vi "Main.vi"(11 "Module Admin":refnum<class "Delacor_lib_QMH_Module Admin.lvclass">) -> ()   [LabVIEW 2020, in "Acquisition.lvlib"]
doc: "This template is based off of the Queued Message Handler design pattern and the Queued Message Handler project template that ships with LabVIEW.\n\nThe main difference is that the queue is private to this module and communication between modules is performed via Broadcast and Request events.\n\nRequest events are wrapped in public API methods and are handled in the Event Handling Loop (EHL) of this VI. Any module can register for Broadcast events sent by this module. The EHL generates messages based on user interface actions.\n\nThe Message Handling Loop (MHL) processes messages generated by the EHL, or by other messages. The messages are string values, so new messages can be added easily to the Message Cases case structure in the MHL. Each message cluster can also provide an optional value for Message Data, which is a variant that can be converted to whatever message-specific data is required.\n_____\nBased on Delacor QMH Project Template 6.0.0.89."
uses:
  Acquisition.lvlib
  <vilib>/Delacor/Delacor QMH/Libraries/Module Admin_class/Delacor_lib_QMH_Module Admin.lvclass
  Module Data--cluster.ctl
  DigitalConfig--cluster.ctl
  AnalogConfig--cluster.ctl
  Stop Argument--cluster.ctl
  <vilib>/Delacor/Delacor QMH/Libraries/Message Queue_class/Delacor_lib_QMH_Message Queue.lvclass/Delacor_lib_QMH_Message Queue.ctl
  <vilib>/Delacor/Delacor QMH/Libraries/Module Admin_class/Delacor_lib_QMH_Module Admin.lvclass/Delacor_lib_QMH_Module Admin.ctl
  Start Acquistion Argument--cluster.ctl
  Set Secuence Argument--cluster.ctl
  <vilib>/Utility/miscctls.llb/LVPointTypeDef.ctl
  <vilib>/DAQmx/read.llb/DAQmx Read (Digital 1D U8 NChan 1Samp).vi
  <vilib>/DAQmx/read.llb/DAQmx Read (Digital 1D Bool NChan 1Samp 1Line).vi
  <vilib>/DAQmx/read.llb/DAQmx Read (Analog 1D Wfm NChan NSamp).vi
  <vilib>/Delacor/Delacor QMH/Libraries/Message Queue_class/Delacor_lib_QMH_Enqueue Message (Single).vi
  <vilib>/Delacor/Delacor QMH/Libraries/Module Admin_class/Delacor_lib_QMH_Get External Launch.vi
  <vilib>/DAQmx/miscellaneous.llb/DAQmx Fill In Error Info.vi
  <vilib>/Utility/error.llb/Error Cluster From Error Code.vi
  <vilib>/ErrorRing/Error Ring.xnode
  <vilib>/Delacor/Delacor QMH/Libraries/Message Queue_class/Delacor_lib_QMH_Message Queue.lvclass
panel:
  out "element":string
  out "error out":errorcluster
  out "Status":string
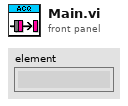
[diagram p1: front panel]
types:
  T1 = typedef "Acquisition.lvlib/Request Events--cluster.ctl" = cluster{"Stop Module":refnum<user-event>, "Show Panel":refnum<user-event>, "Hide Panel":refnum<user-event>, "Get Module Execution Status":refnum<user-event>, "Show Diagram":refnum<user-event>, "Start Acquistion":refnum<user-event>, "WakeUp Digital HL":refnum<user-event>, "WakeUp Analog HL":refnum<user-event>, "Put Analog HL to Sleep":refnum<user-event>, "Put Digital HL to Sleep":refnum<user-event>, "Set Secuence":refnum<user-event>}
  T2 = typedef "Acquisition.lvlib/Module Data--cluster.ctl" = cluster{"Status":string, "DigitalConfig":T3, "AnalogConfig":T4, "ID Max":i32, "Secuence":string[][]}
  T3 = typedef "DigitalConfig--cluster.ctl" = cluster{"Ports/Pins":enum16{"PORTS", "PINS"}, "AcqTime":dbl, "AcqFrecuency":dbl, "Port Digitales":tag[], "Pins":tag[]}
  T4 = typedef "AnalogConfig--cluster.ctl" = cluster{"AcqTime":dbl, "FSamples":dbl, "NSamples":dbl, "Channels":tag[]}
  T5 = enum32{"invalid lock state", "Not Locked", "Locked (No Password)", "Password-protected"}
  T6 = typedef "Acquisition.lvlib/Stop Argument--cluster.ctl" = cluster{"Origin":string, "Exit via Stop Module Req?":bool, "Wait for Module to stop?":bool}
  T7 = typedef "Acquisition.lvlib/Start Acquistion Argument--cluster.ctl" = cluster{"Boolean":bool}
  T8 = typedef "Acquisition.lvlib/Set Secuence Argument--cluster.ctl" = cluster{"ID Max":i32, "Secuence":string[][]}
  T9 = typedef "LVPointTypeDef.ctl" = cluster{"Horizontal":i16, "Vertical":i16}
  T10 = enum32{"Invalid", "Standard", "Closed", "Hidden", "Minimized", "Maximized"}
  T11 = typedef "AcqType--enum.ctl" = enum16{"Digital", "Analog"}
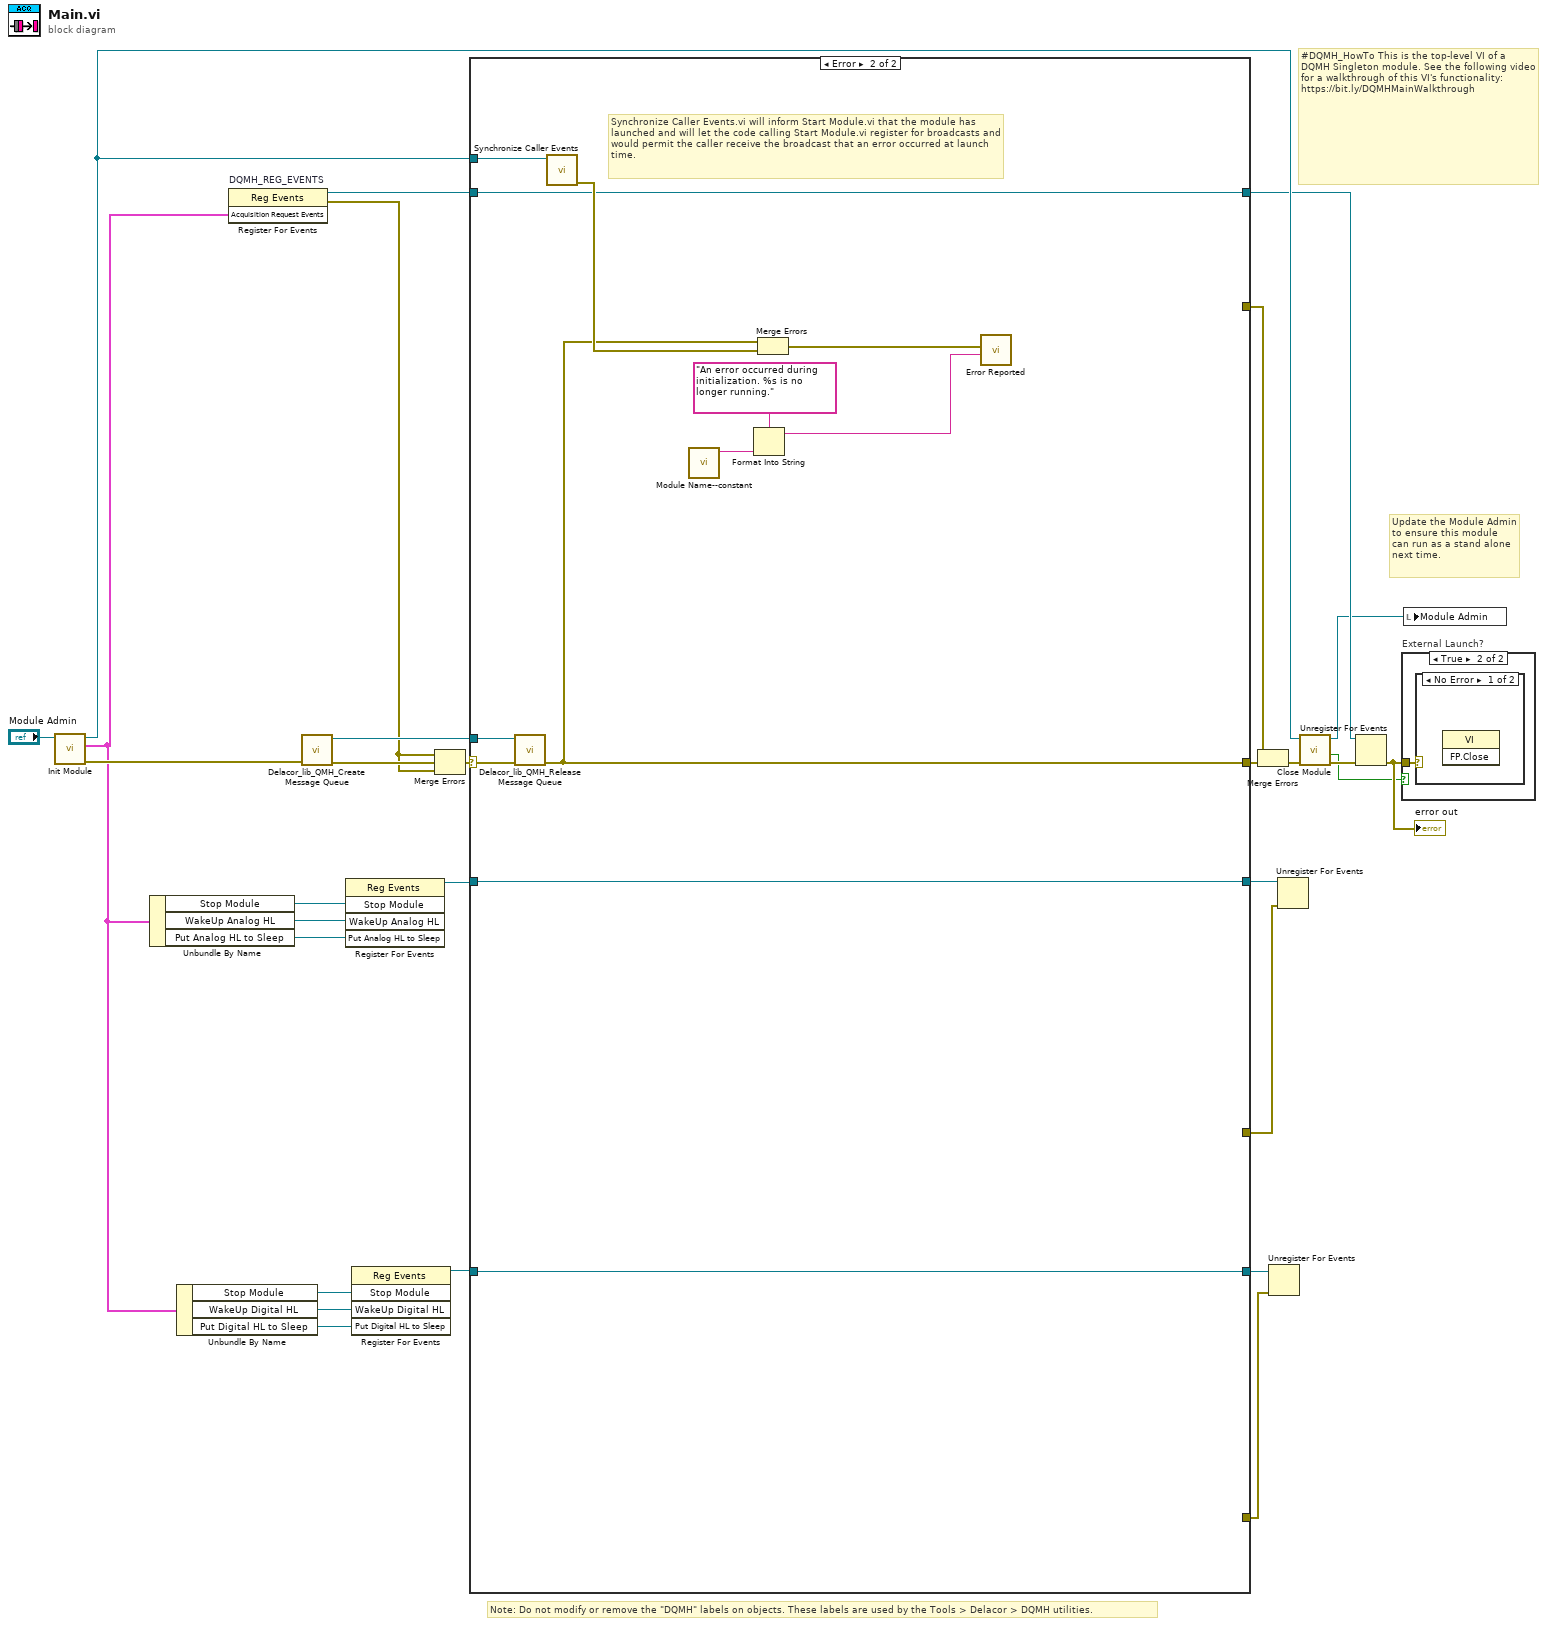
[diagram p0: block diagram]
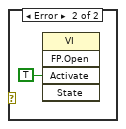
[diagram p3: hidden frame]
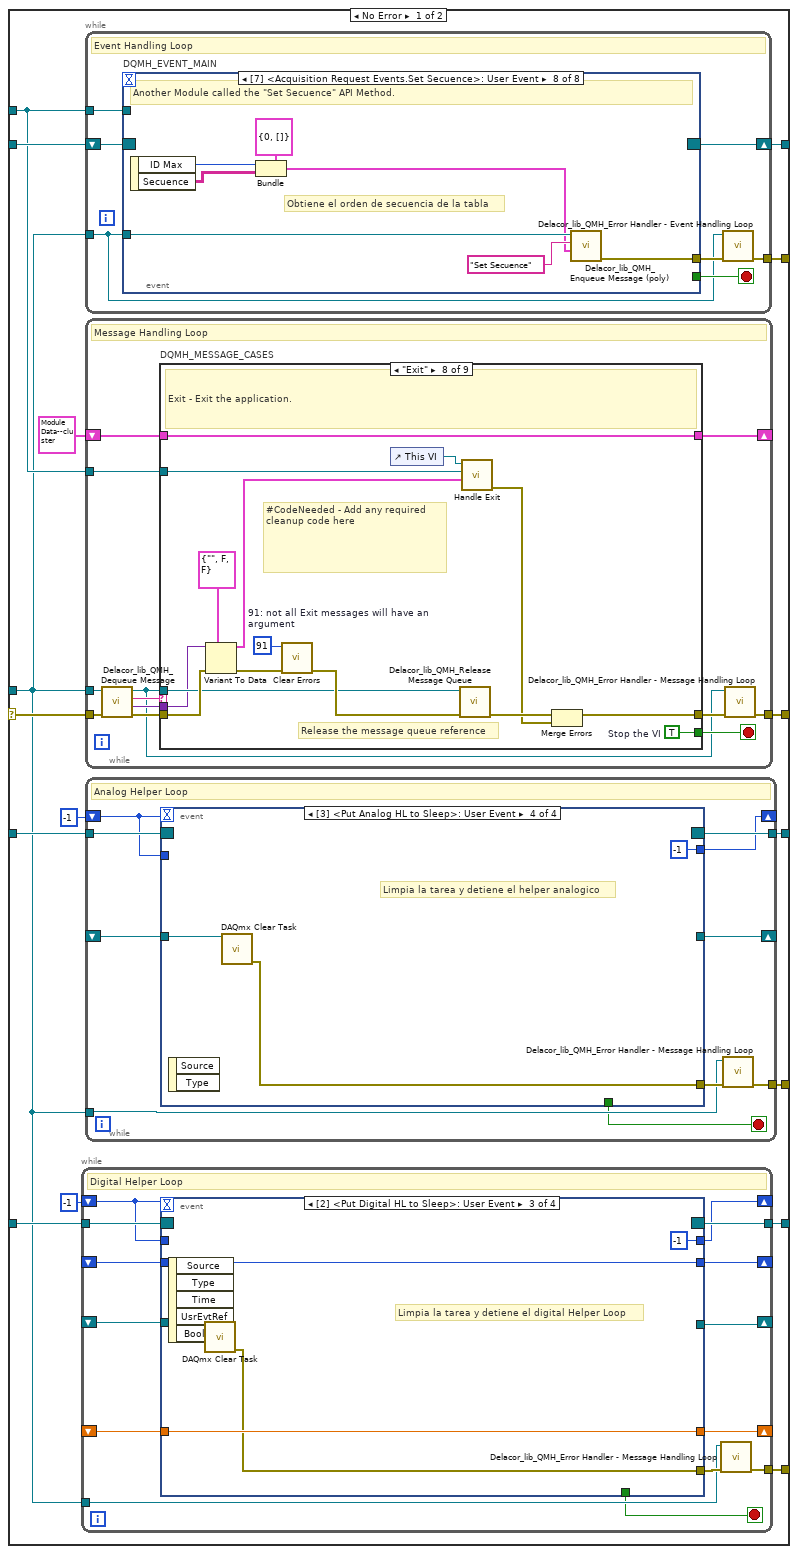
[diagram p4: hidden frame]
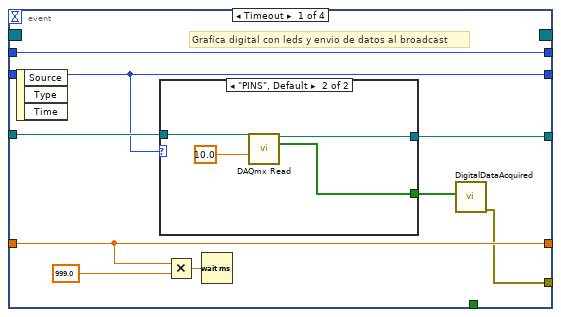
[diagram p5: hidden frame]
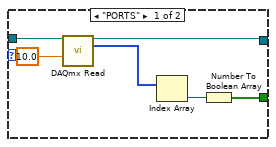
[diagram p6: hidden frame]
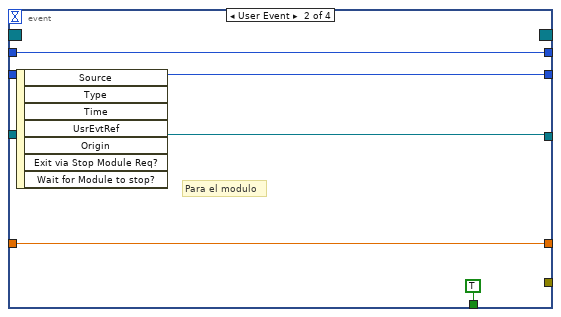
[diagram p7: hidden frame]
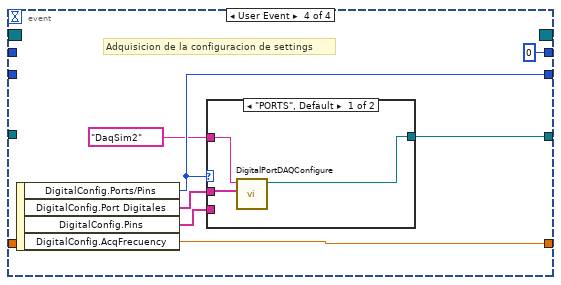
[diagram p8: hidden frame]
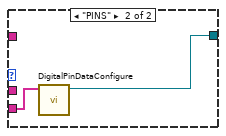
[diagram p9: hidden frame]
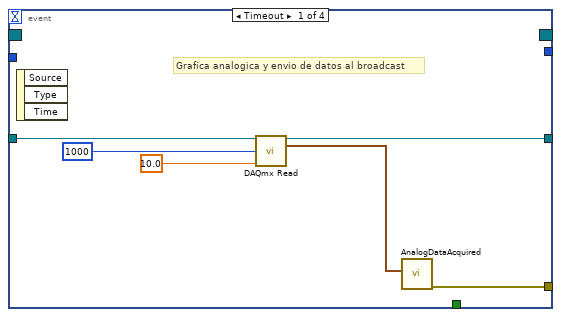
[diagram p10: hidden frame]
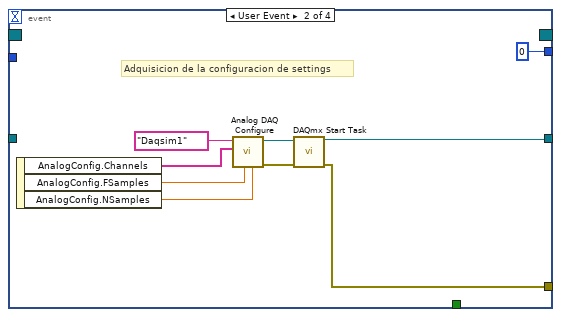
[diagram p11: hidden frame]
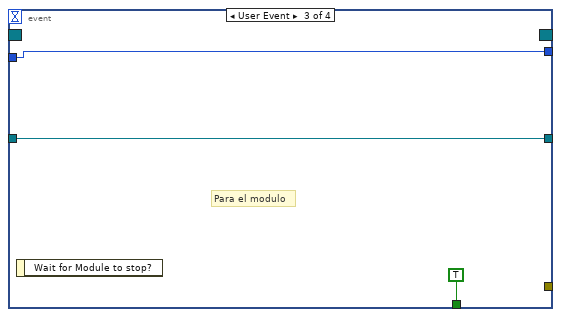
[diagram p12: hidden frame]
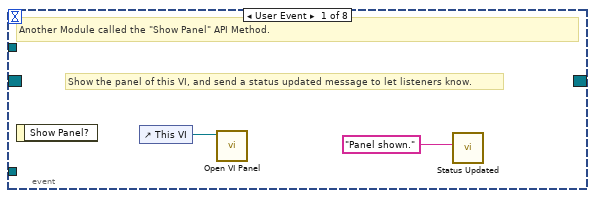
[diagram p13: hidden frame]
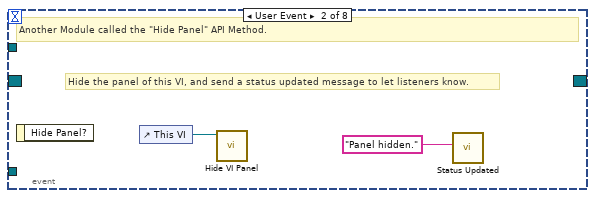
[diagram p14: hidden frame]
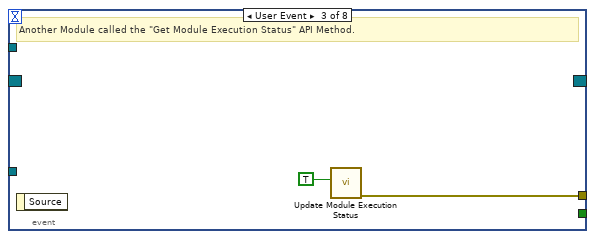
[diagram p15: hidden frame]
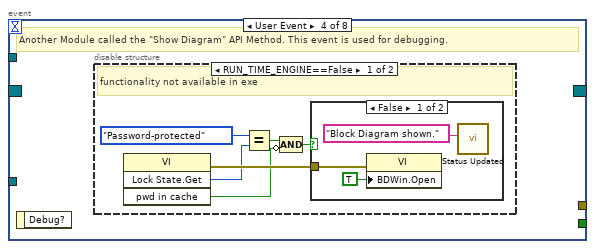
[diagram p16: hidden frame]
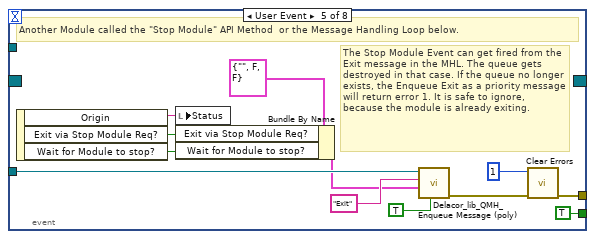
[diagram p19: hidden frame]
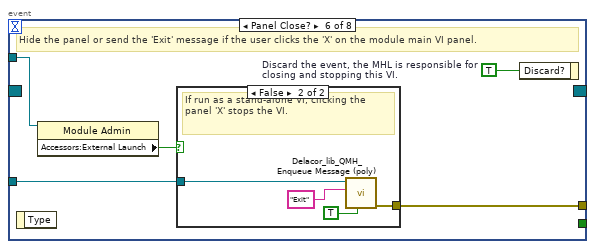
[diagram p20: hidden frame]
diagram:
  # "#DQMH_HowTo This is the top-level VI of a DQMH Singleton module. See the following video for a walkthrough of this VI's functionality: https://bit.ly/DQMHMainWalkthrough"
  # "Note: Do not modify or remove the \"DQMH\" labels on objects. These labels are used by the Tools > Delacor > DQMH utilities."
  # "Update the Module Admin to ensure this module can run as a stand alone next time."
  n1 = call "Init Module.vi"("Singleton Module Admin in"="Module Admin") -> ("error out"=w28:errorcluster, "Acquisition Request Events"=w7:T1, "Singleton Module Admin out"=w21:refnum<class "Delacor_lib_QMH_Module Admin.lvclass">)  [unwired: 8 in]
  n2 = Unbundle By Name(w7) -> ("Stop Module"=w10:refnum<user-event>, "WakeUp Analog HL"=w8:refnum<user-event>, "Put Analog HL to Sleep"=w9:refnum<user-event>)
  n3 = Unbundle By Name(w7) -> ("Stop Module"=w6:refnum<user-event>, "WakeUp Digital HL"=w5:refnum<user-event>, "Put Digital HL to Sleep"=w4:refnum<user-event>)
  n4 = register-events "DQMH_REG_EVENTS"(w7) -> (reference out=w19:refnum<event-registration>, error out=w1:errorcluster)  [unwired: 2 in]
  n5 = call <vilib>:"Delacor_lib_QMH_Create Message Queue.vi"("error in"=w28) -> ("error out"=w23:errorcluster, "Message Queue"=w18:refnum<class "Delacor_lib_QMH_Message Queue.lvclass">)  [unwired: 9 in]
  n6 = register-events(w10, w8, w9) -> (reference out=w12:refnum<event-registration>)  [unwired: 2 in, 1 out]
  n7 = register-events(w6, w5, w4) -> (reference out=w11:refnum<event-registration>)  [unwired: 2 in, 1 out]
  n8 = Merge Errors(w1, w23, w1) -> (w22:errorcluster)
  n9 = case shown="Error" w22 {
    selector: w22 -> [w43 w319]
    tunnel: [w45 w318] -> w29
    tunnel: [w42 w324] -> w20
    tunnel: w19 -> [w40 w324]
    tunnel: w18 -> [w30 w317]
    tunnel: [w44 _] -> w26
    tunnel: w21 -> [w39 w320]
    tunnel: [w38 w316] -> w14
    tunnel: [w37 w315] -> w13
    tunnel: w12 -> [w36 w316]
    tunnel: w11 -> [w35 w315]
    tunnel: [w32 _] -> w3
    tunnel: [w31 _] -> w2
    frame No Error {
      n10 = while {
        tunnel: [w59] -> w37
        tunnel: w35 -> [w58]
        shift-right: [w49] -> _
        shift-left: -1 -> [w57]
        tunnel: [w56] -> w31
        tunnel: w30 -> [w54]
        shift-right: [w52] -> _
        shift-left: _ -> [w53]
        shift-right: [w50] -> _
        shift-left: _ -> [w51]
        shift-right: [w48] -> _
        shift-left: _ -> [w47]
        stop <- w46 stop-if-true
        # "Digital Helper Loop"
        n11 = event shown="[2] <Put Digital HL to Sleep>: User Event" {
          selector: w58 -> [_ _ _ _]
          dyn-events: [_ _ _ _] -> w59
          timeout: w57 -> [_ _ _ _]
          tunnel: w57 -> [w65 w82 _ _]
          tunnel: [w61 _ w84 _] -> w55
          tunnel: w53 -> [w68 w81 w85 _]
          tunnel: [w67 w81 _ w90] -> w52
          tunnel: w51 -> [w63 w80 w86 _]
          tunnel: [w63 w80 w86 w95] -> w50
          tunnel: [w65 w82 -1 0] -> w49
          tunnel: [w60 w83 w88 w93] -> w48
          tunnel: w47 -> [w60 w83 w88 _]
          tunnel: [_ TRUE _ _] -> w46
          event Timeout {
            # "Grafica digital con leds y envio de datos al broadcast"
            n12 = event-data() -> ()  [unwired: 1 in, 3 out]
            n13 = case shown="\"PINS\", Default" w60 {
              tunnel: w68 -> [w74 w78]
              tunnel: [w73 w77] -> w67
              tunnel: [w70 w76] -> w66
              frame "PORTS" {
                n14 = call-poly <vilib>:"DAQmx Read.vi"("task/channels in"=w74, "timeout"=10.0) -> ("task out"=w73:refnum<k21>, "data"=w72:u8[])  [unwired: 11 in, 1 out]
                n15 = Index Array(array=w72) -> (element=w71:u8)  [unwired: 1 in]
                n16 = Number To Boolean Array(number=w71) -> (Boolean array=w70:bool[])
              }
              frame "PINS", Default {
                n17 = call-poly <vilib>:"DAQmx Read.vi"("task/channels in"=w78, "timeout"=10.0) -> ("task out"=w77:refnum<k21>, "data"=w76:bool[])  [unwired: 11 in, 1 out]
              }
            }
            n18 = Multiply(x=w63, y=999.0) -> (x*y=w64:dbl)
            n19 = Wait (ms)(milliseconds to wait=w64) -> ()  [unwired: 1 out]
            n20 = call "DigitalDataAcquired.vi"("DigitalData"=w66) -> ("error out"=w61:errorcluster)  [unwired: 10 in]
          }
          event User Event {
            # "Para el modulo"
            n21 = event-data() -> ()  [unwired: 1 in, 7 out]
          }
          event User Event {
            # "Limpia la tarea y detiene el digital Helper Loop"
            n22 = event-data() -> ()  [unwired: 1 in, 5 out]
            n23 = call <vilib>:"DAQmx Clear Task.vi"("task in"=w85) -> ("error out"=w84:errorcluster)  [unwired: 14 in]
          }
          event User Event {
            # "Adquisicion de la configuracion de settings"
            n24 = event-data() -> ("DigitalConfig.Ports/Pins"=w93:enum16{"PORTS", "PINS"}, "DigitalConfig.Port Digitales"=w92:tag[], "DigitalConfig.Pins"=w89:tag[], "DigitalConfig.AcqFrecuency"=w95:dbl)  [unwired: 1 in]
            n25 = case shown="\"PORTS\", Default" w93 {
              tunnel: w92 -> [w98 _]
              tunnel: tag "DaqSim2" ("DAQmx Device Digital") -> [w97 _]
              tunnel: [w96 w100] -> w90
              tunnel: w89 -> [_ w99]
              frame "PORTS", Default {
                n26 = call "DigitalPortDAQConfigure.vi"("Port Digitales"=w98, "DAQmx Device Digital"=w97) -> ("task out"=w96:refnum<k21>)  [unwired: 8 in, 1 out]
              }
              frame "PINS" {
                n27 = call "DigitalPinDataConfigure.vi"("Pins"=w99) -> ("task out"=w100:refnum<k21>)  [unwired: 9 in, 1 out]
              }
            }
          }
        }
        n28 = call-dynamic "Delacor_lib_QMH_Error Handler - Message Handling Loop.vi"("error in"=w55, "Message Queue in"=w54) -> ("dup error in"=w56:errorcluster)  [unwired: 8 in, 1 out]
      }
      n29 = while {
        tunnel: w30 -> [w132]
        shift-right: [w135] -> w42
        shift-left: w40 -> [w136]
        tunnel: [w137] -> w44
        tunnel: w39 -> [w133]
        stop <- w134 stop-if-true
        # "Event Handling Loop"
        n30 = event "DQMH_EVENT_MAIN" shown="[7] <Acquisition Request Events.Set Secuence>: User Event" {
          selector: w136 -> [_ _ _ _ _ _ _ _]
          dyn-events: [_ _ _ _ _ _ _ _] -> w135
          timeout: _ -> [_ _ _ _ _ _ _ _]
          tunnel: [_ _ _ _ TRUE ("Discard?") _ _ _] -> w134
          tunnel: w132 -> [_ _ _ _ w161 w168 w181 w188]
          tunnel: [_ _ w144 _ w164 w170 w176 w182] -> w138
          tunnel: w133 -> [_ _ _ _ _ w167 _ _]
          event User Event {
            # "Show the panel of this VI, and send a status updated message to let listeners know."
            # "Another Module called the \"Show Panel\" API Method."
            n31 = event-data() -> ()  [unwired: 1 in, 1 out]
            n32 = control-ref of="This VI"() -> (w140:refnum<vi>)
            n33 = call "Open VI Panel.vi"("VI"=w140) -> ()  [unwired: 10 in, 1 out]
            n34 = call "Status Updated.vi"("Status"="Panel shown." ("format string")) -> ()  [unwired: 10 in, 1 out]
          }
          event User Event {
            # "Hide the panel of this VI, and send a status updated message to let listeners know."
            # "Another Module called the \"Hide Panel\" API Method."
            n35 = event-data() -> ()  [unwired: 1 in, 1 out]
            n36 = control-ref of="This VI"() -> (w142:refnum<vi>)
            n37 = call "Hide VI Panel.vi"("VI"=w142) -> ()  [unwired: 10 in, 1 out]
            n38 = call "Status Updated.vi"("Status"="Panel hidden." ("format string")) -> ()  [unwired: 10 in, 1 out]
          }
          event User Event {
            # "Another Module called the \"Get Module Execution Status\" API Method."
            n39 = event-data() -> ()  [unwired: 1 in, 1 out]
            n40 = call "Update Module Execution Status.vi"("Running?"=TRUE) -> ("error out"=w144:errorcluster)  [unwired: 10 in]
          }
          event User Event {
            # "Another Module called the \"Show Diagram\" API Method. This event is used for debugging."
            n41 = event-data() -> ()  [unwired: 1 in, 1 out]
            n42 = disable-structure shown="RUN_TIME_ENGINE==False" {
              frame condition #0 (active) {
                # "functionality not available in exe"
                n43 = invoke class="VI" method="Lock State.Get"() -> (error out=w150:errorcluster, "Get Lock State"=w149:T5, "pwd in cache"=w146:bool)  [unwired: 4 in, 1 out]
                n44 = Equal?(x=T5."Password-protected", y=w149) -> (x = y?=w147:bool)
                n45 = Compound Arithmetic op=AND(w147, invert w146) -> (w145:bool)
                n46 = case shown="False" w145 {
                  tunnel: w150 -> [w153 _]
                  frame False {
                    n47 = property class="VI"(error in=w153, "BDWin.Open"=TRUE ("Block Diagram Window:Open")) -> ()  [unwired: 1 in, 2 out]
                    n48 = call "Status Updated.vi"("Status"="Block Diagram shown." ("format string")) -> ()  [unwired: 10 in, 1 out]
                  }
                  frame True {
                    # "Password-protected VI, and the password is not in the cache. Do not show the diagram."
                  }
                }
              }
              frame condition #1 {
              }
            }
          }
          event User Event {
            # "The Stop Module Event can get fired from the Exit message in the MHL. The queue gets destroyed in that case. If the queue no longer exists, the Enqueue Exit as a priority message will return error 1. It is safe to ignore, because the module is already exiting."
            # "Another Module called the \"Stop Module\" API Method  or the Message Handling Loop below."
            n49 = event-data() -> ("Origin"=w160:string, "Exit via Stop Module Req?"=w156:bool, "Wait for Module to stop?"=w155:bool)  [unwired: 1 in]
            n50 = local write "Status"(w160) -> ()
            n51 = Bundle By Name(cluster=T6 {"Origin"="", "Exit via Stop Module Req?"=FALSE, "Wait for Module to stop?"=FALSE} ("Stop Argument"), "Exit via Stop Module Req?"=w156, "Wait for Module to stop?"=w155) -> (w154:T6)
            n52 = call-poly <vilib>:"Delacor_lib_QMH_Enqueue Message (poly).vi"("Priority Message? (F)"=TRUE, "Message Data"=w154, "Message"="Exit", "Message Queue in"=w161) -> ("error out"=w165:errorcluster)  [unwired: 6 in, 1 out]
            n53 = call <vilib>:"Clear Errors.vi"("error in (no error)"=w165, "specific error code to clear (0: all)"=1) -> ("error out"=w164:errorcluster)  [unwired: 4 in, 1 out]
          }
          event Panel Close? {
            w169 = TRUE  # Discard the event, the MHL is responsible for closing and stopping this VI.
            # "Hide the panel or send the 'Exit' message if the user clicks the 'X' on the module main VI panel."
            n54 = event-data() -> ()  [unwired: 1 in, 1 out]
            n55 = property class="Module Admin"(reference=w167) -> ("Accessors:External Launch"=w166:bool)  [unwired: 1 in, 2 out]
            n56 = case shown="False" w166 {
              tunnel: w168 -> [_ w174]
              tunnel: [_ w175] -> w170
              frame True {
                # "If externally launched, clicking the 'X' hides the panel, but doesn't close it."
                n57 = control-ref of="This VI"() -> (w171:refnum<vi>)
                n58 = call "Hide VI Panel.vi"("VI"=w171) -> ()  [unwired: 10 in, 1 out]
              }
              frame False {
                # "If run as a stand-alone VI, clicking the panel 'X' stops the VI."
                n59 = call-poly <vilib>:"Delacor_lib_QMH_Enqueue Message (poly).vi"("Priority Message? (F)"=TRUE, "Message"="Exit", "Message Queue in"=w174) -> ("error out"=w175:errorcluster)  [unwired: 7 in, 1 out]
              }
            }
            n60 = event-data("Discard?"=w169) -> ()  [unwired: 1 in, 1 out]
          }
          event User Event {
            # "Another Module called the \"Start Acquistion\" API Method."
            n61 = event-data() -> ("Boolean"=w177:bool)  [unwired: 1 in]
            n62 = Bundle(cluster=T7 {"Boolean"=FALSE} ("Start Acquistion Argument"), "Boolean"=w177) -> (w178:T7)
            n63 = call-poly <vilib>:"Delacor_lib_QMH_Enqueue Message (poly).vi"("Message Data"=w178, "Message"="Start Acquistion", "Message Queue in"=w181) -> ("error out"=w176:errorcluster)  [unwired: 7 in, 1 out]
          }
          event User Event {
            # "Obtiene el orden de secuencia de la tabla"
            # "Another Module called the \"Set Secuence\" API Method."
            n64 = event-data() -> ("ID Max"=w184:i32, "Secuence"=w183:string[][])  [unwired: 1 in]
            n65 = Bundle(cluster=T8 {"ID Max"=0, "Secuence"=[]} ("Set Secuence Argument"), "ID Max"=w184, "Secuence"=w183) -> (w185:T8)
            n66 = call-poly <vilib>:"Delacor_lib_QMH_Enqueue Message (poly).vi"("Message Data"=w185, "Message"="Set Secuence", "Message Queue in"=w188) -> ("error out"=w182:errorcluster)  [unwired: 7 in, 1 out]
          }
        }
        n67 = call-dynamic "Delacor_lib_QMH_Error Handler - Event Handling Loop.vi"("error in"=w138, "Message Queue in"=w132) -> ("dup error in"=w137:errorcluster)  [unwired: 8 in, 1 out]
      }
      n68 = while {
        tunnel: w30 -> [w191]
        shift-right: [w195] -> _
        shift-left: T2 {"Status"="", "DigitalConfig"={"Ports/Pins"=enum."PORTS", "AcqTime"=0.0, "AcqFrecuency"=0.0, "Port Digitales"=[], "Pins"=[]}, "AnalogConfig"={"AcqTime"=0.0, "FSamples"=0.0, "NSamples"=0.0, "Channels"=[]}, "ID Max"=0, "Secuence"=[]} ("Data Cluster") -> [w196]
        tunnel: w43 -> [w199]
        tunnel: [w197] -> w45
        tunnel: w39 -> [w189]
        stop <- w194 stop-if-true
        # "Message Handling Loop"
        n69 = call-dynamic "Delacor_lib_QMH_Dequeue Message.vi"("error in"=w199, "Message Queue in"=w191) -> ("error out"=w198:errorcluster, "Message Data"=w192:variant, "Message"=w193:string, "Message Queue out"=w190:refnum<class "Delacor_lib_QMH_Message Queue.lvclass">)  [unwired: 6 in]
        n70 = case "DQMH_MESSAGE_CASES" shown="\"Exit\"" w193 {
          selector: w193 -> [_ _ _ _ _ _ _ _ w302]
          tunnel: w190 -> [_ _ _ _ _ _ w272 w294 _]
          tunnel: w198 -> [w218 w222 w228 w264 w267 w269 w279 w300 w304]
          tunnel: [w216 w222 w228 w263 w266 w269 w275 w297 w305] -> w200
          tunnel: w196 -> [w207 w221 w227 w259 w265 w268 w274 w293 w303]
          tunnel: [w206 w221 w227 w256 w265 w268 w274 w293 w303] -> w195
          tunnel: [_ _ _ _ _ _ _ w292 _] -> w194
          tunnel: w192 -> [_ _ _ w262 _ _ w273 w291 _]
          tunnel: w189 -> [w208 _ _ _ _ _ w271 w286 _]
          frame "Initialize" {
            w202 = "Initial Message" ("Initial Message")
            # "#CodeNeeded - Initialize the appearance of the front panel."
            # "#CodeNeeded - Initialize your state data here."
            # "Initialize - Any operation that needs to be done before the module can receive messages. Synchronize Caller Events.vi will inform Start Module.vi that the module has launched and is ready to receive messages. Module Did Init.vi will broadcast that the module initialized."
            n71 = call "Synchronize Caller Events.vi"("error in (no error)"=w218, "Singleton Module Admin in"=w208) -> ("error out"=w217:errorcluster, "Singleton Module Admin out"=w203:refnum<class "Delacor_lib_QMH_Module Admin.lvclass">)  [unwired: 8 in]
            n72 = property class="Module Admin"(reference=w203) -> ("Accessors:External Launch"=w212:bool)  [unwired: 1 in, 2 out]
            n73 = Select(t=T10."Hidden" ("State"), s=w212, f=T10."Standard" ("State")) -> (s? t:f=w209:T10)
            n74 = call "Module Name--constant.vi"() -> ("Module Name"=w215:string)  [unwired: 11 in]
            n75 = property class="VI"("Front Panel.Title"=w215) -> (reference out=w214:refnum<vi>, error out=w220:errorcluster)  [unwired: 2 in]
            n76 = call "Module Name--constant.vi"() -> ("Module Name"=w204:string)  [unwired: 11 in]
            n77 = invoke class="VI" method="FP.Open"(reference=w214, error in=w220, "State"=w209) -> (reference out=w213:refnum<vi>, error out=w219:errorcluster)  [unwired: 2 in, 3 out]
            n78 = Bundle By Name(cluster=w207, "Status"=w202) -> (w206:T2)
            n79 = call "Module Did Init.vi"("error in (no error)"=w217, "Initialized?"=TRUE, "Origin"=w204) -> ("error out"=w216:errorcluster)  [unwired: 8 in]
            n80 = invoke class="VI" method="FP.Center"(reference=w213, error in=w219) -> ()  [unwired: 1 in, 3 out]
            n81 = property on="Pane" class="Pane"("Origin"=T9 {"Horizontal"=0, "Vertical"=0}) -> ()  [unwired: 2 in, 2 out]
            "Status" <- w202
          }
          frame "---Module Specific---" {
            # "Separator -- The following cases handle messages specific to this Module."
          }
          frame "Start Acquistion" {
            # "Mando la secuencia cada que pasa el tiempo descrito en settings"
            # "Start Acquistion"
            n82 = Unbundle By Name(w227) -> ("ID Max"=w223:i32, "Secuence"=w225:string[][])
            n83 = Increment(x=w223) -> (x+1=w224:i32)
            n84 = for {
              N: w224 -> [_]
              shift-right: [w243] -> _
              shift-left: 0 -> [w241]
              tunnel: w225 -> [w242]
              # "Broadcast con el tipo \nde ACQ"
              n85 = Index Array(array=w242, index (row)=w241) -> (element=w238:string[])  [unwired: 1 in]
              n86 = Increment(x=w241) -> (x+1=w243:i32)
              n87 = Index Array(array=w238, index #1=1 ("index"), index #2=6 ("index")) -> (element #1=w237:string, element #2=w236:string)
              "element" <- w237
              n88 = Empty String/Path?(string/path=w236) -> (empty?=w229:bool)
              n89 = call "TypeAcq.vi"("TypeAcqName"=w237) -> ()  [unwired: 10 in, 1 out]
              n90 = call "TestSecuence.vi"("String"=w237, "Result Set"=w238) -> ("Time"=w233:i32, "ACQType"=w232:T11, "AnalogConfig"=w230:T4, "DigitalConfig"=w231:T3)  [unwired: 6 in]
              n91 = case shown="\"Digital\", Default" w232 {
                tunnel: w231 -> [w245 _]
                tunnel: w230 -> [_ w255]
                tunnel: w229 -> [w246 _]
                frame "Digital", Default {
                  n92 = case shown="False" w246 {
                    tunnel: w245 -> [w249 w253]
                    tunnel: [w250 w252] -> w244
                    frame False {
                      n93 = Bundle By Name(cluster=w249, "Ports/Pins"=enum16{"PORTS", "PINS"}."PORTS") -> (w250:T3)
                    }
                    frame True {
                      n94 = Bundle By Name(cluster=w253, "Ports/Pins"=enum16{"PORTS", "PINS"}."PINS") -> (w252:T3)
                    }
                  }
                  n95 = call "WakeUp Digital HL.vi"("DigitalConfig"=w244, "Digital TimeOut"=0) -> ()  [unwired: 9 in, 1 out]
                }
                frame "Analog" {
                  n96 = call "WakeUp Analog HL.vi"("AnalogConfig"=w255, "Analog TimeOut"=0) -> ()  [unwired: 9 in, 1 out]
                }
              }
              n97 = Multiply(x=w233, y=1000.0) -> (x*y=w235:dbl)
              n98 = Wait (ms)(milliseconds to wait=w235) -> ()  [unwired: 1 out]
              n99 = call "Put Digital HL to Sleep.vi"() -> ()  [unwired: 11 in, 1 out]
              n100 = call "Put Analog HL to Sleep.vi"() -> ()  [unwired: 11 in, 1 out]
            }
          }
          frame "Set Secuence" {
            # "Subo la secuencia"
            # "Set Secuence"
            n101 = Variant To Data(error in=w264, type=T8 {"ID Max"=0, "Secuence"=[]} ("Set Secuence Argument"), Variant=w262) -> (data=w260:T8, error out=w263:errorcluster)
            n102 = Unbundle By Name(w260) -> ("ID Max"=w257:i32, "Secuence"=w258:string[][])
            n103 = Bundle By Name(cluster=w259, "ID Max"=w257, "Secuence"=w258) -> (w256:T2)
          }
          frame "---Copy This Frame---" {
            # "Duplicate this frame when creating new messages.  Change this comment in the duplicated frame to describe this message."
            n104 = Merge Errors(w267) -> (w266:errorcluster)
          }
          frame "---Exit and Error Handling---" {
            # "Separator - The following cases handle errors and exit messages."
          }
          frame "Error" {
            # "#CodeRecommended - If you ever change the name of this \"Error\" message, you'll need to update the name in the Check Loop Error.vi as well."
            # "#CodeRecommended - If the module is running in standalone mode (External Launch = FALSE), this code will pop up an error dialog and call the 'Exit' message if an error occurs. Add more fine-grained error handling here."
            # "Error - Check the error message data and respond accordingly. This message is sent by the \"Error Handler\" VIs at the end of each loop in this application."
            n105 = property class="Module Admin"(reference=w271) -> ("Accessors:External Launch"=w270:bool)  [unwired: 1 in, 2 out]
            n106 = Variant To Data(error in=w279, type=errorcluster {"status"=FALSE, "code"=0, "source"=""} ("error constant"), Variant=w273) -> (data=w280:errorcluster, error out=w277:errorcluster)
            n107 = call "Error Reported.vi"("Error"=w280) -> ()  [unwired: 10 in, 1 out]
            n108 = case shown="False" w270 {
              tunnel: [w285 _] -> w276
              tunnel: w272 -> [w283 _]
              tunnel: w280 -> [w284 _]
              frame False {
                # "If the module is running standalone, then pop up an error dialog and call the \"Exit\" message."
                n109 = call <vilib>:"Simple Error Handler.vi"("error in (no error)"=w284) -> ()  [unwired: 4 in, 5 out]
                n110 = call-poly <vilib>:"Delacor_lib_QMH_Enqueue Message (poly).vi"("Priority Message? (F)"=TRUE, "Message"="Exit", "Message Queue in"=w283) -> ("error out"=w285:errorcluster)  [unwired: 7 in, 1 out]
              }
              frame True {
                # "If the module was launched externally, calling the Error Reported broadcast VI is the only action performed by the \"Error\" message. The module's caller can then process the error appropriately."
              }
            }
            n111 = Merge Errors(w277, w276) -> (w275:errorcluster)
            n112 = local write "error out"(w275) -> ()
          }
          frame "Exit" {
            w290 = 91  # 91: not all Exit messages will have an argument
            w292 = TRUE  # Stop the VI
            # "Release the message queue reference"
            # "#CodeNeeded - Add any required cleanup code here"
            # "Exit - Exit the application."
            n113 = Variant To Data(error in=w300, type=T6 {"Origin"="", "Exit via Stop Module Req?"=FALSE, "Wait for Module to stop?"=FALSE} ("Stop Argument"), Variant=w291) -> (data=w288:T6, error out=w296:errorcluster)
            n114 = call <vilib>:"Clear Errors.vi"("error in (no error)"=w296, "specific error code to clear (0: all)"=w290) -> ("error out"=w299:errorcluster)  [unwired: 4 in, 1 out]
            n115 = control-ref of="This VI"() -> (w287:refnum<vi>)
            n116 = call-dynamic "Delacor_lib_QMH_Release Message Queue.vi"("error in"=w299, "Message Queue"=w294) -> ("error out"=w298:errorcluster)  [unwired: 9 in]
            n117 = call "Handle Exit.vi"("Stop Argument"=w288, "Admin in"=w286, "VI reference"=w287) -> ("error out"=w295:errorcluster)  [unwired: 7 in, 1 out]
            n118 = Merge Errors(w298, w295) -> (w297:errorcluster)
          }
          frame Default {
            # "'Default' case only runs if there is a message that isn't defined in any of the other cases.  Output a programming error."
            n119 = call "Module Name--constant.vi"() -> ("Module Name"=w301:string)  [unwired: 11 in]
            n120 = xnode "Error Ring"("parameter 0"=w302, "parameter 1"=w301) -> ("error out"=w306:errorcluster)
            n121 = Merge Errors(w304, w306) -> (w305:errorcluster)
          }
        }
        n122 = call-dynamic "Delacor_lib_QMH_Error Handler - Message Handling Loop.vi"("error in"=w200, "Message Queue in"=w190) -> ("dup error in"=w197:errorcluster)  [unwired: 8 in, 1 out]
      }
      n123 = while {
        tunnel: [w110] -> w38
        tunnel: w36 -> [w109]
        shift-right: [w102] -> _
        shift-left: -1 -> [w108]
        shift-right: [w106] -> _
        shift-left: _ -> [w107]
        tunnel: w30 -> [w104]
        tunnel: [w103] -> w32
        stop <- w101 stop-if-true
        # "Analog Helper Loop"
        n124 = event shown="[3] <Put Analog HL to Sleep>: User Event" {
          selector: w109 -> [_ _ _ _]
          dyn-events: [_ _ _ _] -> w110
          timeout: w108 -> [_ _ _ _]
          tunnel: w108 -> [_ _ w127 _]
          tunnel: w107 -> [w116 _ w128 w131]
          tunnel: [w115 w117 w128 _] -> w106
          tunnel: [w111 w118 _ w130] -> w105
          tunnel: [_ 0 w127 -1] -> w102
          tunnel: [_ _ TRUE _] -> w101
          event Timeout {
            # "Grafica analogica y envio de datos al broadcast"
            n125 = event-data() -> ()  [unwired: 1 in, 3 out]
            n126 = call-poly <vilib>:"DAQmx Read.vi"("task/channels in"=w116, "number of samples per channel"=1000, "timeout"=10.0) -> ("task out"=w115:refnum<k21>, "data"=w112:waveform(dbl)[])  [unwired: 10 in, 1 out]
            n127 = call "AnalogDataAcquired.vi"("AnalogData"=w112) -> ("error out"=w111:errorcluster)  [unwired: 10 in]
          }
          event User Event {
            # "Adquisicion de la configuracion de settings"
            n128 = event-data() -> ("AnalogConfig.Channels"=w123:tag[], "AnalogConfig.FSamples"=w122:dbl, "AnalogConfig.NSamples"=w121:dbl)  [unwired: 1 in]
            n129 = call "Analog DAQ Configure.vi"("number of samples"=w121, "rate"=w122, "Canales"=w123, "DAQ Board Name"=tag "Daqsim1") -> ("error out"=w119:errorcluster, "task out"=w120:refnum<k21>)  [unwired: 6 in]
            n130 = call <vilib>:"DAQmx Start Task.vi"("task/channels in"=w120, "error in"=w119) -> ("task out"=w117:refnum<k21>, "error out"=w118:errorcluster)  [unwired: 12 in]
          }
          event User Event {
            # "Para el modulo"
            n131 = event-data() -> ()  [unwired: 1 in, 1 out]
          }
          event User Event {
            # "Limpia la tarea y detiene el helper analogico"
            n132 = event-data() -> ()  [unwired: 1 in, 2 out]
            n133 = call <vilib>:"DAQmx Clear Task.vi"("task in"=w131) -> ("error out"=w130:errorcluster)  [unwired: 14 in]
          }
        }
        n134 = call-dynamic "Delacor_lib_QMH_Error Handler - Message Handling Loop.vi"("error in"=w105, "Message Queue in"=w104) -> ("dup error in"=w103:errorcluster)  [unwired: 8 in, 1 out]
      }
    }
    frame Error {
      # "Synchronize Caller Events.vi will inform Start Module.vi that the module has launched and will let the code calling Start Module.vi register for broadcasts and would permit the caller receive the broadcast that an error occurred at launch time."
      n135 = call-dynamic "Delacor_lib_QMH_Release Message Queue.vi"("error in"=w319, "Message Queue"=w317) -> ("error out"=w318:errorcluster)  [unwired: 9 in]
      n136 = call "Synchronize Caller Events.vi"("Singleton Module Admin in"=w320) -> ("error out"=w325:errorcluster)  [unwired: 9 in, 1 out]
      n137 = call "Module Name--constant.vi"() -> ("Module Name"=w323:string)  [unwired: 11 in]
      n138 = Format Into String(format string="An error occurred during initialization. %s is no longer running.", w323) -> (resulting string=w321:string)  [unwired: 2 in, 1 out]
      n139 = Merge Errors(w318, w325) -> (w326:errorcluster)
      n140 = call "Error Reported.vi"("Additional Information"=w321, "Error"=w326) -> ()  [unwired: 9 in, 1 out]
    }
  }
  n141 = Merge Errors(w26, w29) -> (w25:errorcluster)
  n142 = Unregister For Events(event registration refnum=w13, error in=w2) -> ()  [unwired: 1 out]
  n143 = Unregister For Events(event registration refnum=w14, error in=w3) -> ()  [unwired: 1 out]
  n144 = call "Close Module.vi"("error in (no error)"=w25, "Module Admin in"=w21) -> ("error out"=w27:errorcluster, "External Launch"=w15:bool, "Module Admin out"=w16:refnum<class "Delacor_lib_QMH_Module Admin.lvclass">)  [unwired: 7 in]
  n145 = Unregister For Events(event registration refnum=w20, error in=w27) -> (error out=w24:errorcluster)
  "error out" <- w24
  n146 = case "External Launch?" shown="True" w15 {
    tunnel: w24 -> [_ w327]
    frame False {
    }
    frame True {
      n147 = case shown="No Error" w327 {
        frame No Error {
          n148 = invoke class="VI" method="FP.Close"() -> ()  [unwired: 3 in, 3 out]
        }
        frame Error {
          n149 = invoke class="VI" method="FP.Open"("Activate"=TRUE ("Activate?")) -> ()  [unwired: 4 in, 5 out]
        }
      }
    }
  }
  n150 = local write "Module Admin"(w16) -> ()
